vi "Update Tool Status.vi"(6 "wait for reply (T)":bool=TRUE, 8 "error in (no error)":errorcluster) -> (0 "error out":errorcluster, 1 "timed out?":bool, 2 "Reply Payload":T1)   [LabVIEW 2015, in "Tool Module.lvlib"]
doc: "<b>Note</b>: This VI was renamed by the DQMH Rename Event utility. Make sure the VI Description is updated to reflect the new event name, then delete this comment.\n\nGet the current data from the Motion Status Reader. This is an asynchronous retreival at the rate for updating the tool status to the caller.\n_____\nCreated using Delacor QMH Event Scripter 4.2.1.88."
uses:
  Tool Module.lvlib
  Update Tool Status (Reply Payload)--cluster.ctl
  Update Motion Status Argument--cluster.ctl
  _Motion Status Reader SM enum--typedef.ctl
  Update Tool Status Argument--cluster.ctl
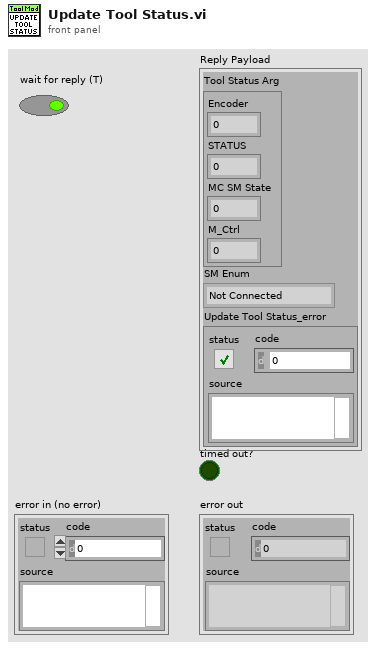
[diagram p1: front panel]
types:
  T1 = typedef "Tool Module.lvlib/Update Tool Status (Reply Payload)--cluster.ctl" = cluster{"Tool Status Arg":T2, "SM Enum":T3, "Update Tool Status_error":errorcluster}
  T2 = typedef "Tool Module.lvlib/Update Motion Status Argument--cluster.ctl" = cluster{"Encoder":i32, "STATUS":u16, "MC SM State":u16, "M_Ctrl":u16}
  T3 = typedef "Tool Module.lvlib/_Motion Status Reader SM enum--typedef.ctl" = enum16{"Not Connected", "Connect", "Idle", "Receive Data", "Disconnect"}
  T4 = typedef "Tool Module.lvlib/Update Tool Status Argument--cluster.ctl" = cluster{"Wait Notifier":refnum<notifier>, "wait for reply":bool}
  T5 = typedef "Tool Module.lvlib/Request Events--cluster.ctl" = cluster{"Stop Module":refnum<user-event>, "Show Panel":refnum<user-event>, "Hide Panel":refnum<user-event>, "Get Module Execution Status":refnum<user-event>, "Show Diagram":refnum<user-event>, "Test Trig 2":refnum<user-event>, "GOTO":refnum<user-event>, "Start Inspect":refnum<user-event>, "CONNECT":refnum<user-event>, "Get All Inspect Data":refnum<user-event>, "Get Inspection Limits":refnum<user-event>, "Set Inspection Limits":refnum<user-event>, "Update Motion Status":refnum<user-event>, "Start Data Monitor":refnum<user-event>, "Get FPGA Setup Params":refnum<user-event>, "Set FPGA Setup Params":refnum<user-event>, "Set Tool Config":refnum<user-event>, "Get Tool Config":refnum<user-event>, "Set Integration Count":refnum<user-event>, "Set Laser Params":refnum<user-event>, "Get Mtrl Ctrl Reg":refnum<user-event>, "Commit Ctrl Reg":refnum<user-event>, "Set Event Logger":refnum<user-event>, "Write to File":refnum<user-event>, "Read from File":refnum<user-event>, "Set Device Temp Thresholds":refnum<user-event>, "Get Cycle Count":refnum<user-event>, "Return FPGA Setup Data":refnum<user-event>, "Update FPGA Setup Data":refnum<user-event>, "Setup Timer 1":refnum<user-event>, "Setup Timer 2":refnum<user-event>, "Tool Status Reader Cmd":refnum<user-event>, "Update Tool Status":refnum<user-event>}
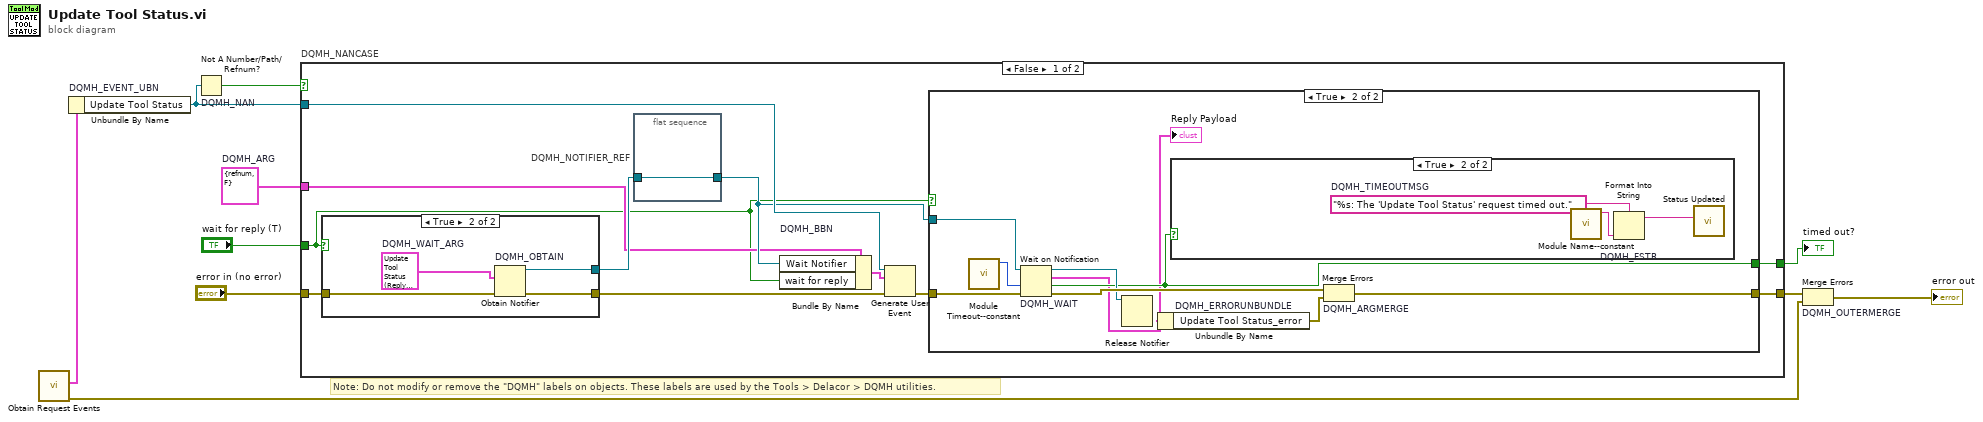
[diagram p0: block diagram]
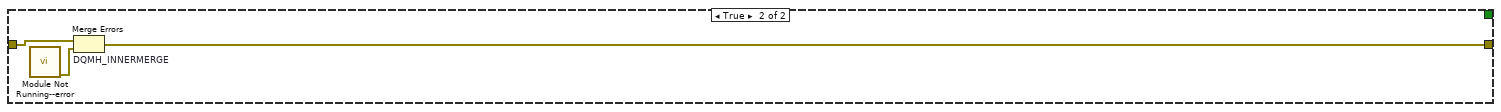
[diagram p5: hidden frame]
diagram:
  w4 = T4 {"Wait Notifier"=refnum, "wait for reply"=FALSE}  # DQMH_ARG
  # "Note: Do not modify or remove the \"DQMH\" labels on objects. These labels are used by the Tools > Delacor > DQMH utilities."
  n1 = call "Obtain Request Events.vi"() -> ("error out"=w2:errorcluster, "Tool Module Request Events"=w1:T5)  [unwired: 10 in]
  n2 = Unbundle By Name "DQMH_EVENT_UBN"(w1) -> ("Update Tool Status"=w8:refnum<user-event>)
  n3 = Not A Number/Path/Refnum? "DQMH_NAN"(number/path/refnum=w8) -> (NaN/Path/Refnum?=w7:bool)
  n4 = case "DQMH_NANCASE" shown="False" w7 {
    tunnel: "error in (no error)" -> [w21 w43]
    tunnel: w8 -> [w19 _]
    tunnel: [w16 w42] -> w5
    tunnel: [w17 _] -> w6
    tunnel: w4 -> [w12 _]
    tunnel: "wait for reply (T)" -> [w11 _]
    frame False {
      n5 = case shown="True" w11 {
        tunnel: w21 -> [w36 w40]
        tunnel: [w36 w39] -> w18
        tunnel: [_ w37] -> w14
        frame False {
        }
        frame True {
          w38 = T1 {"Tool Status Arg"={"Encoder"=0, "STATUS"=0, "MC SM State"=0, "M_Ctrl"=0}, "SM Enum"=enum."Not Connected", "Update Tool Status_error"={"status"=FALSE, "code"=0, "source"=""}}  # DQMH_WAIT_ARG
          n6 = Obtain Notifier "DQMH_OBTAIN"(notification data type=w38, error in (no error)=w40) -> (notifier out=w37:refnum<notifier>, error out=w39:errorcluster)  [unwired: 2 in, 1 out]
        }
      }
      n7 = flat-sequence "DQMH_NOTIFIER_REF" {
        tunnel: w14 -> [w22]
        tunnel: [w22] -> w13
        frame #0 {
        }
      }
      n8 = Bundle By Name "DQMH_BBN"(cluster=w12, "Wait Notifier"=w13, "wait for reply"=w11) -> (w15:T4)
      n9 = Generate User Event(user event=w19, event data cluster=w15, error in=w18) -> (error out=w20:errorcluster)  [unwired: 1 in, 1 out]
      n10 = case shown="True" w11 {
        tunnel: w20 -> [w23 w32]
        tunnel: w13 -> [_ w30]
        tunnel: [_ w28] -> w17
        tunnel: [w23 w27] -> w16
        frame False {
        }
        frame True {
          n11 = call "Module Timeout--constant.vi"() -> ("Module Timeout"=w24:i32)  [unwired: 11 in]
          n12 = Wait on Notification "DQMH_WAIT"(notifier=w30, timeout in ms (-1)=w24, error in (no error)=w32) -> (notifier out=w29:refnum<notifier>, notification=w25:T1, timed out?=w28:bool, error out=w31:errorcluster)  [unwired: 1 in]
          "Reply Payload" <- w25
          n13 = Release Notifier(notifier=w29) -> ()  [unwired: 2 in, 3 out]
          n14 = Unbundle By Name "DQMH_ERRORUNBUNDLE"(w25) -> ("Update Tool Status_error"=w26:errorcluster)
          n15 = case shown="True" w28 {
            frame False {
            }
            frame True {
              w35 = "%s: The 'Update Tool Status' request timed out."  # DQMH_TIMEOUTMSG
              n16 = call "Module Name--constant.vi"() -> ("Module Name"=w34:string)  [unwired: 11 in]
              n17 = Format Into String "DQMH_FSTR"(format string=w35, w34) -> (resulting string=w33:string)  [unwired: 2 in, 1 out]
              n18 = call "Status Updated.vi"("Status"=w33) -> ()  [unwired: 10 in, 1 out]
            }
          }
          n19 = Merge Errors "DQMH_ARGMERGE"(w31, w26) -> (w27:errorcluster)
        }
      }
    }
    frame True {
      n20 = call "Module Not Running--error.vi"() -> ("error out"=w41:errorcluster)  [unwired: 11 in]
      n21 = Merge Errors "DQMH_INNERMERGE"(w43, w41) -> (w42:errorcluster)
    }
  }
  "timed out?" <- w6
  n22 = Merge Errors "DQMH_OUTERMERGE"(w5, w2) -> (→"error out":errorcluster)
